vi "MGI Set Plot Names (Chart).vi"(7 "Set Plot Legend Height? (T)":bool=TRUE, 8 "error in (no error)":errorcluster, 10 "Plot Name[]":string[](array[string]), 11 "Chart Ref":refnum<vi>) -> (0 "error out":errorcluster, 3 "Chart Ref (out)":refnum<vi>)   [LabVIEW 2020]
doc: "Sets the plot names as specified, optionally growing the Plot Legend to fit the number of names. If Plot Name[] is empty, then the Plot Legend is hidden, otherwise it is shown.\n\nAuthored by Shawn D. Walpole\nsupport@mooregoodideas.com\nwww.mooregoodideas.com\n\nCopyright (c) 2010, Moore Good Ideas, Inc.\n\nAll rights reserved.\n\nRedistribution and use in source and binary forms, with or without modification, are permitted provided that the following conditions are met:\n\n * Redistributions of source code must retain the above copyright notice, this list of conditions and the following disclaimer.\n * Redistributions in binary form must reproduce the above copyright notice, this list of conditions and the following disclaimer in the documentation and/or other materials provided with the distribution.\n * Neither the name of Moore Good Ideas, Inc. nor the names of its contributors may be used to endorse or promote products derived from this software without specific prior written permission.\n\nTHIS SOFTWARE IS PROVIDED BY THE COPYRIGHT HOLDERS AND CONTRIBUTORS \"AS IS\" AND ANY EXPRESS OR IMPLIED WARRANTIES, INCLUDING, BUT NOT LIMITED TO, THE IMPLIED WARRANTIES OF MERCHANTABILITY AND FITNESS FOR A PARTICULAR PURPOSE ARE DISCLAIMED. IN NO EVENT SHALL THE COPYRIGHT OWNER OR CONTRIBUTORS BE LIABLE FOR ANY DIRECT, INDIRECT, INCIDENTAL, SPECIAL, EXEMPLARY, OR CONSEQUENTIAL DAMAGES (INCLUDING, BUT NOT LIMITED TO, PROCUREMENT OF SUBSTITUTE GOODS OR SERVICES; LOSS OF USE, DATA, OR PROFITS; OR BUSINESS INTERRUPTION) HOWEVER CAUSED AND ON ANY THEORY OF LIABILITY, WHETHER IN CONTRACT, STRICT LIABILITY, OR TORT (INCLUDING NEGLIGENCE OR OTHERWISE) ARISING IN ANY WAY OUT OF THE USE OF THIS SOFTWARE, EVEN IF ADVISED OF THE POSSIBILITY OF SUCH DAMAGE."
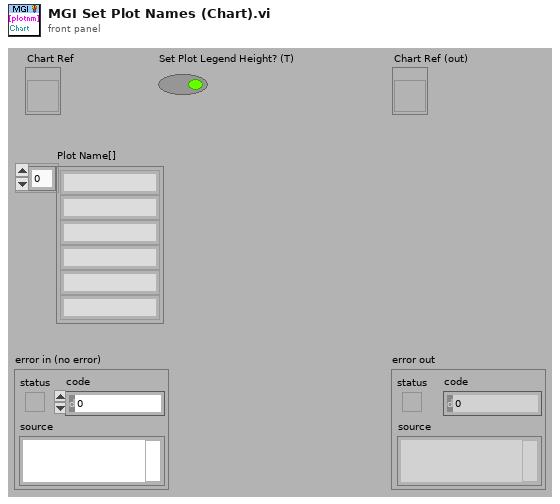
[diagram p1: front panel]
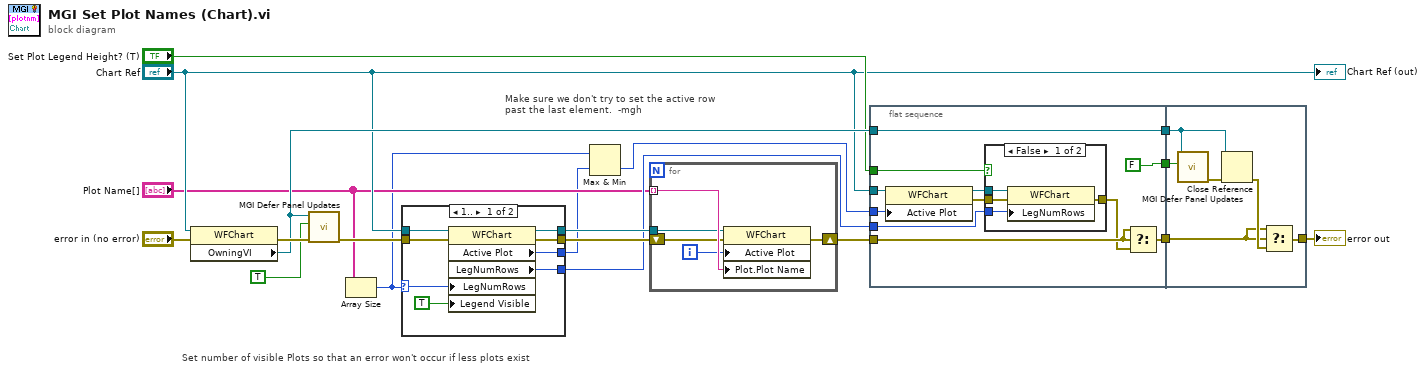
[diagram p0: block diagram]
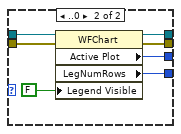
[diagram p2: hidden frame]
diagram:
  # "Make sure we don't try to set the active row \npast the last element.  -mgh"
  # "Set number of visible Plots so that an error won't occur if less plots exist"
  n1 = property on="Property Node" class="WFChart"(reference="Chart Ref", error in="error in (no error)") -> (error out=w14:errorcluster, "OwningVI"=w9:refnum<vi>)  [unwired: 1 out]
  n2 = call <userlib>:"MGI Defer Panel Updates.vi"("Error In"=w14, "Defer Updates?"=TRUE ("Defer Updates? (False: Restore state)"), "VI Reference (Caller)"=w9) -> ("Error Out"=w11:errorcluster)  [unwired: 8 out]
  n3 = Array Size(array="Plot Name[]") -> (size(s)=w1:i32)
  n4 = case shown="1.." w1 {
    selector: w1 -> [w21 _]
    tunnel: [w27 w34] -> w19
    tunnel: [w26 w33] -> w3
    tunnel: [w25 w32] -> w18
    tunnel: "Chart Ref" -> [w24 w31]
    tunnel: w11 -> [w23 w30]
    tunnel: [w22 w29] -> w7
    frame 1.. {
      n5 = property on="Property Node" class="WFChart"(reference=w24, error in=w23, "LegNumRows"=w21, "Legend Visible"=TRUE ("Legend:Visible")) -> (reference out=w27:refnum<vi>, error out=w25:errorcluster, "Active Plot"=w26:u32, "LegNumRows"=w22:u32)
    }
    frame ..0 {
      n6 = property on="Property Node" class="WFChart"(reference=w31, error in=w30, "Legend Visible"=FALSE ("Legend:Visible")) -> (reference out=w34:refnum<vi>, error out=w32:errorcluster, "Active Plot"=w33:u32, "LegNumRows"=w29:u32)
    }
  }
  n7 = Max & Min(x=w1, y=w3) -> (min(x,y)=w2:u32)  [unwired: 1 out]
  n8 = for {
    tunnel: "Plot Name[]" -> [w39] mode=indexing
    tunnel: w19 -> [w37]
    shift-right: [w35] -> w17
    shift-left: w18 -> [w36]
    i -> [w38]
    n9 = property on="Property Node" class="WFChart"(reference=w37, error in=w36, "Active Plot"=w38, "Plot.Plot Name"=w39) -> (error out=w35:errorcluster)  [unwired: 1 out]
  }
  n10 = flat-sequence {
    tunnel: w2 -> [w50]
    tunnel: "Chart Ref" -> [w49]
    tunnel: w17 -> [w48]
    tunnel: [w47] -> w12
    tunnel: [w46] -> w10
    tunnel: w9 -> [w46]
    tunnel: [FALSE] -> w8
    tunnel: w7 -> [w41]
    tunnel: "Set Plot Legend Height? (T)" -> [w40]
    tunnel: [w58] -> w16
    tunnel: w12 -> [w59]
    tunnel: w10 -> [w57]
    tunnel: w8 -> [w56]
    frame #0 {
      n11 = property on="Property Node" class="WFChart"(reference=w49, "Active Plot"=w50) -> (reference out=w43:refnum<vi>, error out=w44:errorcluster)  [unwired: 1 in]
      n12 = case shown="False" w40 {
        tunnel: w44 -> [w54 w55]
        tunnel: w43 -> [w53 _]
        tunnel: [w52 w55] -> w42
        tunnel: w41 -> [w51 _]
        frame False {
          n13 = property on="Property Node" class="WFChart"(reference=w53, error in=w54, "LegNumRows"=w51) -> (error out=w52:errorcluster)  [unwired: 1 out]
        }
        frame True {
        }
      }
      n14 = Select(t=w48, s=w48, f=w42) -> (s? t:f=w47:errorcluster)
    }
    frame #1 {
      n15 = call <userlib>:"MGI Defer Panel Updates.vi"("Defer Updates?"=w56, "VI Reference (Caller)"=w57) -> ("Error Out"=w61:errorcluster)  [unwired: 1 in, 8 out]
      n16 = Close Reference(reference=w57, error in (no error)=w61) -> (error out=w60:errorcluster)
      n17 = Select(t=w59, s=w59, f=w60) -> (s? t:f=w58:errorcluster)
    }
  }
  "Chart Ref (out)" <- "Chart Ref"
  "error out" <- w16
